vi "PWM Generator.vi"(10 "Period":u32, 11 "Active Time":u32) -> (3 "Output":bool)   [LabVIEW 2012, in "MyFPGACode.lvlib"]
doc: "This VI will generate a PWM signal with the specified Duty Cycle and Period. Each period consists of a active state followed by an incactive state.\n\nThis VI is marked as re-entrant so that it it can be placed multiple times on the block diagram. Each time this VI is dropped on the block diagram, duplicate logic will be created in the FPGA.\n\nThis subVI was designed to work within a single cycle timed loop. If it is not used inside a single cycle timed loop, care should be taken to ensure that this VI is called at regular intervals. The period and duty cycle will be in terms of this interval period.\n\n<B>Inputs:</B>\n<B>Active Time</B> - This is the active pulse width in terms of ticks if using in a single cycle timed loop or in terms of what ever interval it is called at. If the Duty cylce is equal to or greater than then the period the output will remain in it's active state. If the duty cycle is set to 0, the output will remain in it's inactive state. The duty cycle will only be reloaded at the end of each period.\n\n<B>Period</B> - This is the length of one coplete Active/ Inactive pulse cycle. The period will only be reloaded at the end of each period. A period of 0 is equal to a period of 1.\n\n<B>Outputs:</B>\n<B>Output</B> - This is the output state of the PWM generator. A TRUE indicates the active state, a FALSE indicates the inactive state."
uses:
  MyFPGACode.lvlib
panel:
  out "Curr. Duty Cycle":u32
  out "Curr. Period":u32
  out "Period Count":u32
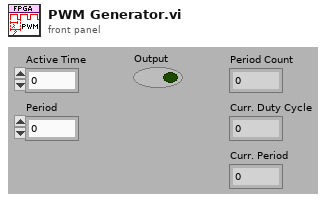
[diagram p1: front panel]
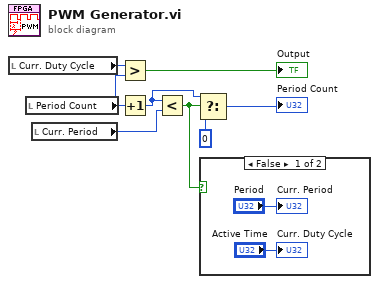
[diagram p0: block diagram]
diagram:
  n1 = local read "Curr. Duty Cycle"() -> (w3:u32)
  n2 = local read "Period Count"() -> (w7:u32)
  n3 = local read "Curr. Period"() -> (w2:u32)
  n4 = Greater?(x=w3, y=w7) -> (0:→"Output":bool)
  n5 = Increment(x=w7) -> (x+1=w6:u32)
  n6 = Less?(x=w6, y=w2) -> (x < y?=w1:bool)
  n7 = Select(t=w6, s=w1, f=u32 0 ("t")) -> (s? t:f=→"Period Count":u32)
  n8 = case shown="False" w1 {
    frame False {
      "Curr. Period" <- "Period"
      "Curr. Duty Cycle" <- "Active Time"
    }
    frame True {
    }
  }
